vi "Default--constant.vi"(8 "error in":errorcluster, 11 "Generator in":refnum<class "GeneradorAmplificado.lvclass">) -> (0 "error out":errorcluster, 3 "Generator out":refnum<class "GeneradorAmplificado.lvclass">)   [LabVIEW 2020, in "FGen.lvlib" / "GeneradorAmplificado.lvclass"]
uses:
  GeneradorAmplificado.lvclass
  C:/Users/DELL/Documents/GitClones/Labview/IVJoshua2P-/Libraries/FGen/Generador/Generador.lvclass
  Generador/Generador.lvclass/Generador.ctl
  Generador/Set amplitude.vi
  Generador/Set frequency.vi
  Generador/Set offset.vi
  Generador/Set phase.vi
  Generador/Set sampling info.vi
  Generador/Set square wave duty cycle (%).vi
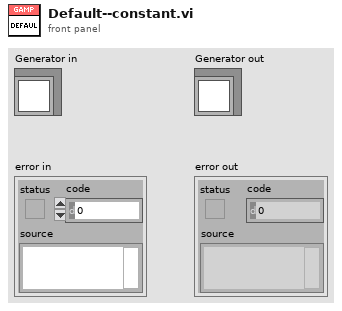
[diagram p1: front panel]
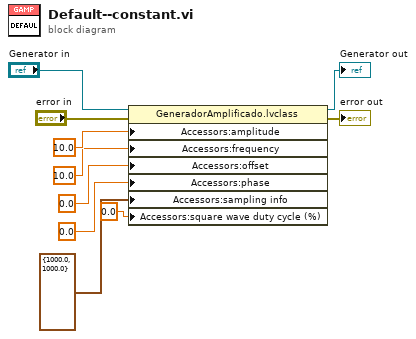
[diagram p0: block diagram]
diagram:
  n1 = property class="GeneradorAmplificado.lvclass"(reference="Generator in", error in="error in", "Accessors:amplitude"=10.0 ("amplitude"), "Accessors:frequency"=10.0 ("frequency"), "Accessors:offset"=0.0 ("offset"), "Accessors:phase"=0.0 ("phase"), "Accessors:sampling info"=cluster{"Fs":dbl, "s":dbl} {"Fs"=1000.0, "s"=1000.0} ("sampling info"), "Accessors:square wave duty cycle (%)"=0.0 ("square wave duty cycle (%)")) -> (reference out=→"Generator out":refnum<class "GeneradorAmplificado.lvclass">, error out=→"error out":errorcluster)
